vi "Launch.vi"() -> ()   [LabVIEW 2024]
uses:
  TesterModule/TesterModule.lvclass
  C:/Github/JQMH/JQMHCore/Module/JQMHModule.lvclass
  <vilib>/Analysis/baseanly.llb/Mean (DBL).vi
  JQMHCore/Module/JQMHModule.lvclass
  <vilib>/Analysis/NI_AALBase.lvlib
panel:
  out "x-y":dbl format="%#_6p"
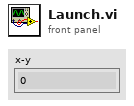
[diagram p1: front panel]
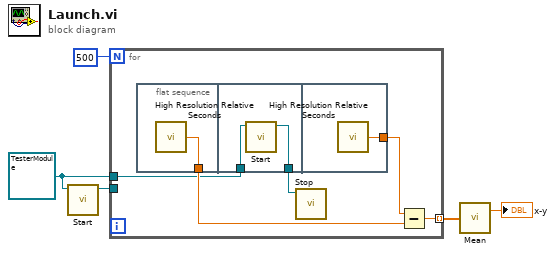
[diagram p0: block diagram]
diagram:
  w2 = refnum<class "TesterModule.lvclass"> refnum ("TesterModule.lvclass")
  n1 = call "Start.vi"("JQMHCore in"=w2) -> ("JQMHCore out"=w1:refnum<class "JQMHModule.lvclass">)  [unwired: 9 in, 1 out]
  n2 = for {
    N: 500 -> [_]
    tunnel: [w8] -> w5 mode=indexing
    tunnel: w2 -> [w7]
    tunnel: w1 -> [_]
    n3 = flat-sequence {
      tunnel: [w11] -> w9
      tunnel: w7 -> [w13]
      tunnel: [w12] -> w6
      tunnel: [w14] -> w10
      frame #0 {
        n4 = call <vilib>:"High Resolution Relative Seconds.vi"() -> ("relative seconds"=w11:dbl)
      }
      frame #1 {
        n5 = call "Start.vi"("JQMHCore in"=w13) -> ("JQMHCore out"=w12:refnum<class "JQMHModule.lvclass">)  [unwired: 9 in, 1 out]
      }
      frame #2 {
        n6 = call <vilib>:"High Resolution Relative Seconds.vi"() -> ("relative seconds"=w14:dbl)
      }
    }
    n7 = call "Stop.vi"("JQMHCore in"=w6) -> ()  [unwired: 9 in, 2 out]
    n8 = Subtract(x=w10, y=w9) -> (x-y=w8:dbl)
  }
  n9 = call-poly <vilib>:"Mean.vi"("X"=w5) -> ("mean"=→"x-y":dbl)  [unwired: 1 out]
